vi "TemperatureReader.vi"() -> ()   [LabVIEW 2017]
uses:
  <vilib>/Utility/config.llb/Read Key (String).vi
  <vilib>/Instr/_visa.llb/VISA Configure Serial Port (Instr).vi
  <vilib>/Utility/config.llb/NI_LVConfig.lvlib
panel:
  in  "s to wait":u32=1000
  in  "stop":bool
  out "trimmed string":string
  in  "ComPort":refnum<visa-resource-name>
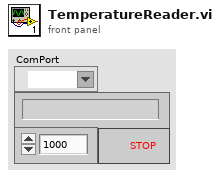
[diagram p1: front panel]
types:
  T1 = enum16{"open", "replace", "create", "open or create", "replace or create", "replace or create with confirmation"}
  T2 = typedef "NI_LVConfig.lvlib/Config Data RefNum.ctl" = refnum<k1>
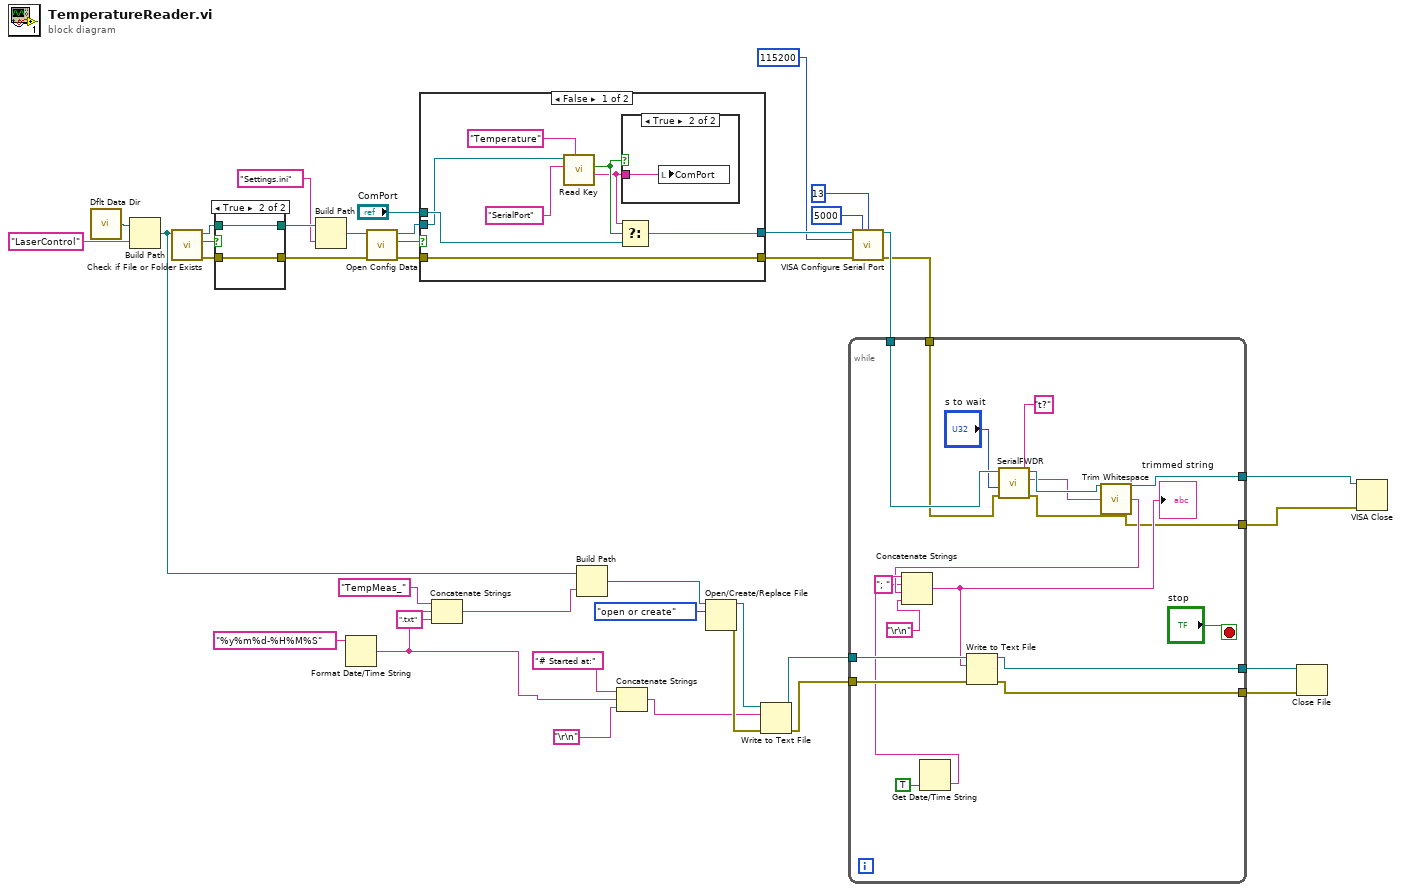
[diagram p0: block diagram]
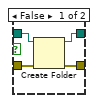
[diagram p4: hidden frame]
diagram:
  n1 = call <vilib>:"Dflt Data Dir.vi"() -> ("App:Default Data Directory"=w39:path)
  n2 = Build Path(base path=w39, name or relative path="LaserControl") -> (appended path=w15:path)
  n3 = call <vilib>:"Check if File or Folder Exists.vi"("path"=w15) -> ("error out"=w34:errorcluster, "file or folder exists?"=w36:bool, "dup path"=w35:path)  [unwired: 8 in]
  n4 = case shown="True" w36 {
    tunnel: [w42 w45] -> w32
    tunnel: w35 -> [w43 w45]
    tunnel: w34 -> [w41 w44]
    tunnel: [w40 w44] -> w33
    frame False {
      n5 = Create Folder(path (use dialog)=w43, error in=w41) -> (created path=w42:path, error out=w40:errorcluster)  [unwired: 1 in, 1 out]
    }
    frame True {
    }
  }
  n6 = Build Path(base path=w32, name or relative path="Settings.ini") -> (appended path=w37:path)
  n7 = Format Date/Time String(time format string (%c)="%y%m%d-%H%M%S") -> (date/time string=w3:string)  [unwired: 2 in]
  n8 = call <vilib>:"Open Config Data.vi"("error in (no error)"=w33, "configuration file path"=w37) -> ("error out"=w30:errorcluster, "file created?"=w27:bool, "refnum"=w28:T2)  [unwired: 7 in]
  n9 = case shown="False" w27 {
    tunnel: "ComPort" -> [w50 w56]
    tunnel: w30 -> [w49 w55]
    tunnel: w28 -> [w46 _]
    tunnel: [w49 w55] -> w22
    tunnel: [w48 w56] -> w26
    frame False {
      n10 = call-poly <vilib>:"Read Key.vi"("section"="Temperature", "key"="SerialPort", "refnum"=w46) -> ("value"=w51:string, "found?"=w52:bool)  [unwired: 5 in, 2 out]
      n11 = Select(t=w51, s=w52, f=w50) -> (s? t:f=w48:string)
      n12 = case shown="True" w52 {
        tunnel: w51 -> [_ w54]
        frame False {
        }
        frame True {
          n13 = local write "ComPort"(w54) -> ()
        }
      }
    }
    frame True {
    }
  }
  n14 = Concatenate Strings("TempMeas_" ("name or relative path"), w3, ".txt" ("string")) -> (w1:string)
  n15 = Build Path(base path=w15, name or relative path=w1) -> (appended path=w14:path)
  n16 = Concatenate Strings("# Started at:" ("string"), w3, "\r\n") -> (w8:string)
  n17 = Open/Create/Replace File(file path (use dialog)=w14, operation (0:open)=T1."open or create") -> (refnum out=w11:refnum<file>, error out=w13:errorcluster)  [unwired: 4 in, 1 out]
  n18 = Write to Text File(file (use dialog)=w11, text=w8, error in=w13) -> (refnum out=w10:refnum<file>, error out=w12:errorcluster)  [unwired: 1 in, 1 out]
  n19 = call-poly "VISA Configure Serial Port"("VISA resource name"=w26, "timeout (10sec)"=u32 5000, "termination char\n(0xA = '\\n' = LF)"=u8 13 ("termination char\n(0xA = '\\n' = LF)"), "baud rate (9600)"=u32 115200, "error in (no error)"=w22) -> ("VISA resource name out"=w21:refnum<visa-resource-name>, "error out"=w20:errorcluster)  [unwired: 9 in]
  n20 = while {
    tunnel: w21 -> [w63]
    tunnel: w20 -> [w61]
    tunnel: [w62] -> w19
    tunnel: [w60] -> w18
    tunnel: w10 -> [w73]
    tunnel: [w72] -> w17
    tunnel: [w71] -> w16
    tunnel: w12 -> [w70]
    stop <- "stop" stop-if-true
    n21 = Get Date/Time String(want seconds? (F)=TRUE) -> (time string=w68:string)  [unwired: 2 in, 1 out]
    n22 = call "SerialFWDR.vi"("error in (no error)"=w61, "Delay Time (s)"="s to wait", "CommandString"="t?", "VISA Refnum in"=w63) -> ("error out"=w60:errorcluster, "trimmed string"=w59:string, "VISA Refnum out"=w62:refnum<visa-resource-name>)  [unwired: 5 in]
    n23 = call <vilib>:"Trim Whitespace.vi"("string"=w59) -> ("trimmed string"=w66:string)  [unwired: 1 in]
    n24 = Concatenate Strings(w68, "; " ("string"), w66, "\r\n") -> (w69:string)
    "trimmed string" <- w69
    n25 = Write to Text File(file (use dialog)=w73, text=w69, error in=w70) -> (refnum out=w72:refnum<file>, error out=w71:errorcluster)  [unwired: 1 in, 1 out]
  }
  n26 = Close File(refnum=w17, error in=w16) -> ()  [unwired: 2 out]
  n27 = VISA Close(VISA resource name=w19, error in (no error)=w18) -> ()  [unwired: 1 out]
